vi "Crop Zero.vi"(2 "Paired data":sgl[](array[numeric]), 3 "Search data":sgl[](array[numeric])) -> (0 "Paired data out":sgl[](array[numeric]), 1 "Searched data out":sgl[](array[numeric]))   [LabVIEW 2014]
doc: "Takes a 1D arrays and removes the 0s and then removes the corresponding entries from a second array (optional)"
panel:
  # "Remove any 0 entries from the search data and the mathcing data"
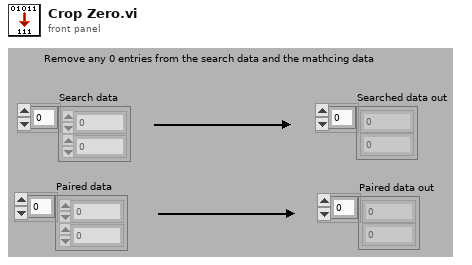
[diagram p1: front panel]
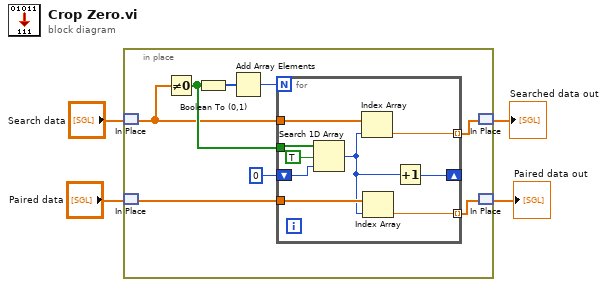
[diagram p0: block diagram]
diagram:
  n1 = in-place {
    n2 = in-place-match #1("Search data") -> (w8:sgl[])
    n3 = in-place-match #2("Paired data") -> (w6:sgl[])
    n4 = Not Equal To 0?(x=w8) -> (x != 0?=w10:bool[])
    n5 = Boolean To (0,1)(Boolean=w10) -> (0, 1=w12:i16[])
    n6 = Add Array Elements(numeric array=w12) -> (sum=w11:i16)
    n7 = for {
      N: w11 -> [_]
      tunnel: w10 -> [w17]
      tunnel: w8 -> [w21]
      tunnel: [w20] -> w7 mode=indexing
      tunnel: [w19] -> w5 mode=indexing
      tunnel: w6 -> [w18]
      shift-right: [w14] -> _
      shift-left: 0 -> [w15]
      n8 = Search 1D Array(1D array=w17, element=TRUE, start index (0)=w15) -> (index of element=w13:i32)
      n9 = Index Array(array=w21, index=w13) -> (element=w20:sgl)
      n10 = Index Array(array=w18, index=w13) -> (element=w19:sgl)
      n11 = Increment(x=w13) -> (x+1=w14:i32)
    }
    n12 = in-place-match #1(w7) -> (→"Searched data out":sgl[])
    n13 = in-place-match #2(w5) -> (→"Paired data out":sgl[])
  }
